vi "util-serial-init.vi"(10 "NewVal":refnum<visa-resource-name>, 11 "Port":refnum<visa-resource-name>) -> (0 "error out":errorcluster)   [LabVIEW 2024]
uses:
  controls/enum.io-interface.ctl
  controls/typePathSelector.ctl
  controls/ini-key.ctl
  <vilib>/Utility/libraryn.llb/Create Directory Recursive.vi
  <vilib>/Utility/config.llb/Write Key (String).vi
  <vilib>/Utility/config.llb/NI_LVConfig.lvlib
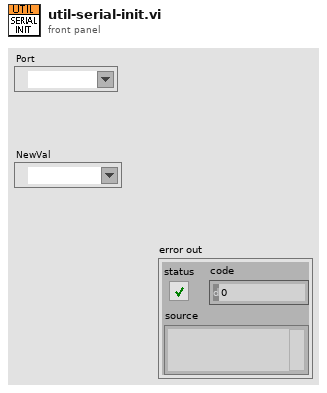
[diagram p1: front panel]
types:
  T1 = typedef "ini-key.ctl" = enum16{"INI.PROJECT_NAME", "INI.ENV", "INI.ENG.SERIAL", "INI.ENG.INTERVAL_MS", "INI.LOCAL.LONGITUDE", "INI.LOCAL.LATITUDE", "INI.LOCAL.TIMEZONE"}
  T2 = typedef "typePathSelector.ctl" = enum16{"DIR_PROCS", "DIR_CONFIG", "DIR_TEMPLATE", "DIR_IO_FILE", "DIR_RECORD", "DIR_LOG", "DIR_RUNTIME", "DIR_PRESET", "DIR_INI"}
  T3 = typedef "enum.io-interface.ctl" = enum16{"IO_VISA_WR-RD", "IO_VISA_OPEN", "IO_VISA_CLOSE", "IO_VISA_CLEAR"}
  T4 = typedef "NI_LVConfig.lvlib/Config Data RefNum.ctl" = refnum<k1>
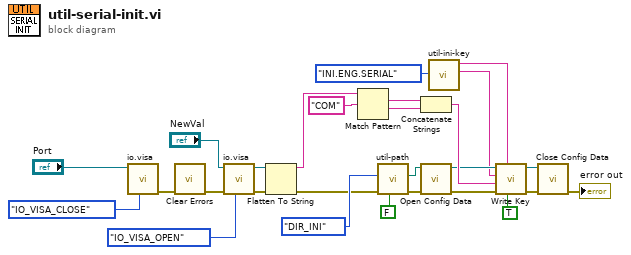
[diagram p0: block diagram]
diagram:
  n1 = call "io.visa.vi"("operation in (wr-rd)"=enum.io-interface."IO_VISA_CLOSE", "VISA Refnum in"="Port") -> ("error out"=w16:errorcluster)  [unwired: 6 in, 3 out]
  n2 = call <vilib>:"Clear Errors.vi"("error in (no error)"=w16) -> ("error out"=w15:errorcluster)  [unwired: 5 in, 1 out]
  n3 = call "io.visa.vi"("operation in (wr-rd)"=enum.io-interface."IO_VISA_OPEN", "error in (no error)"=w15, "VISA Refnum in"="NewVal") -> ("error out"=w21:errorcluster, "VISA Refnum out"=w22:refnum<visa-resource-name>)  [unwired: 5 in, 2 out]
  n4 = Flatten To String(anything=w22, error in (no error)=w21) -> (data string=w23:string, error out=w5:errorcluster)  [unwired: 2 in, 1 out]
  n5 = Match Pattern(string=w23, regular expression="COM") -> (match substring=w26:string, after substring=w25:string)  [unwired: 1 in, 2 out]
  n6 = call "util-path.vi"("Create Folders?(F)"=FALSE, "error in"=w5, "Selected Folder (PROCS)"=typePathSelector."DIR_INI" ("Selected Folder (PROCEDURE_DIR)")) -> ("error out"=w7:errorcluster, "SelectedPath"=w9:path)  [unwired: 4 in, 3 out]
  n7 = Concatenate Strings(w26, w25) -> (w27:string)
  n8 = call <vilib>:"Open Config Data.vi"("error in (no error)"=w7, "configuration file path"=w9) -> ("error out"=w8:errorcluster, "refnum"=w10:T4)  [unwired: 7 in, 1 out]
  n9 = call "util-ini-key.vi"("key"=ini-key."INI.ENG.SERIAL" ("input 1")) -> ("key"=w1:string, "section"=w2:string)  [unwired: 9 in]
  n10 = call-poly <vilib>:"Write Key.vi"("write raw string? (F)"=TRUE, "section"=w2, "error in (no error)"=w8, "value"=w27, "key"=w1, "refnum"=w10) -> ("error out"=w13:errorcluster, "refnum out"=w14:T4)  [unwired: 3 in, 1 out]
  n11 = call <vilib>:"Close Config Data.vi"("error in (no error)"=w13, "refnum"=w14) -> ("error out"=→"error out":errorcluster)  [unwired: 8 in, 1 out]
